vi "GDSError_MergeError.vi"(0 "error in 1":errorcluster, 1 "error in 2":errorcluster, 2 "Error Array":errorcluster[](array[cluster]), 8 "Display a DialogBox?":bool) -> (14 "error out":errorcluster, 16 "All Error Out":errorcluster[](array[cluster]))   [LabVIEW 2020]
doc: "Söker efter error i inkommande errorcluster.\nLetar först i Error 1 sedan Error 2, sist Error Array."
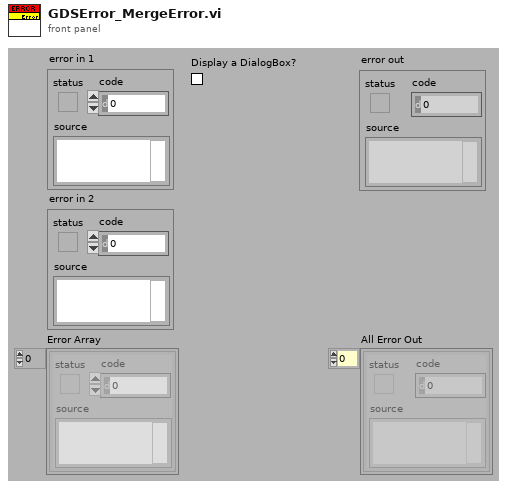
[diagram p1: front panel]
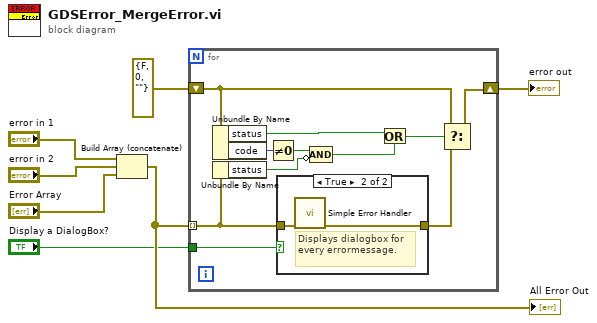
[diagram p0: block diagram]
diagram:
  n1 = Build Array (concatenate)("error in 1", "error in 2", "Error Array") -> (w2:errorcluster[])
  "All Error Out" <- w2
  n2 = for {
    tunnel: w2 -> [w12] mode=indexing
    shift-right: [w18] -> w7
    shift-left: errorcluster {"status"=FALSE, "code"=0, "source"=""} ("error out") -> [w9]
    tunnel: "Display a DialogBox?" -> [w8]
    n3 = Unbundle By Name(w9) -> ("status"=w11:bool, "code"=w13:i32)
    n4 = Unbundle By Name(w12) -> ("status"=w14:bool)
    n5 = Not Equal To 0?(x=w13) -> (x != 0?=w15:bool)
    n6 = case shown="True" w8 {
      tunnel: [w19 w21] -> w17
      tunnel: w12 -> [w19 w20]
      frame False {
      }
      frame True {
        # "Displays dialogbox for every errormessage."
        n7 = call <vilib>:"Simple Error Handler.vi"("error in (no error)"=w20) -> ("error out"=w21:errorcluster)  [unwired: 4 in, 4 out]
      }
    }
    n8 = Compound Arithmetic op=AND(w15, invert w14) -> (w16:bool)
    n9 = Or(x=w11, y=w16) -> (x .or. y?=w10:bool)
    n10 = Select(t=w9, s=w10, f=w17) -> (s? t:f=w18:errorcluster)
  }
  "error out" <- w7
